vi "Read PID SP Lim.vi"(8 "error in (no error)":errorcluster, 11 "HE_reg in":refnum<class "HE_reg.lvclass">) -> (0 "error out":errorcluster, 2 "PID SP Limiter":refnum<class "PID SP Limiter.lvclass">, 3 "HE_reg out":refnum<class "HE_reg.lvclass">)   [LabVIEW 2019, in "Heating.lvlib" / "HE_reg.lvclass"]
uses:
  HE_reg.lvclass
  Reg/PID/PID SP Limiter/PID SP Limiter.lvclass
  HE_reg.lvclass/HE_reg.ctl
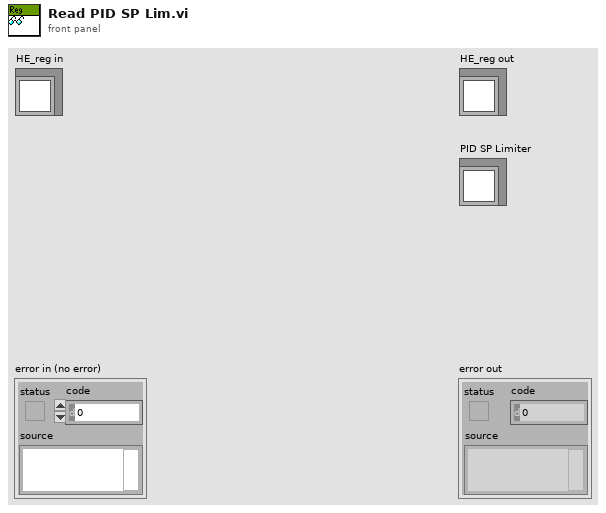
[diagram p1: front panel]
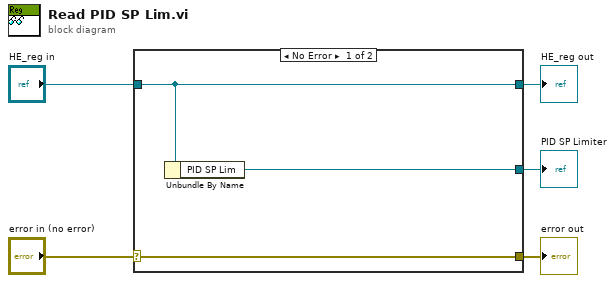
[diagram p0: block diagram]
diagram:
  n1 = case shown="No Error" "error in (no error)" {
    selector: "error in (no error)" -> [w8 w9]
    tunnel: [w8 w9] -> w4
    tunnel: [w7 w10] -> w2
    tunnel: "HE_reg in" -> [w7 w10]
    tunnel: [w6 _] -> w1
    frame No Error {
      n2 = Unbundle By Name(w7) -> ("PID SP Lim"=w6:refnum<class "PID SP Limiter.lvclass">)
    }
    frame Error {
    }
  }
  "error out" <- w4
  "HE_reg out" <- w2
  "PID SP Limiter" <- w1
